vi "write relay.vi"(8 "error in (no error)":errorcluster, 9 "value":bool, 10 "index":i32, 11 "USB DAQ in":refnum<class "USB DAQ.lvclass">) -> (0 "error out":errorcluster, 3 "USB DAQ out":refnum<class "USB DAQ.lvclass">)   [LabVIEW 2025, in "USB DAQ.lvclass"]
uses:
  USB DAQ.lvclass
  USB DAQ.lvclass/USB DAQ.ctl
  <vilib>/DAQmx/write.llb/DAQmx Write (Digital 1D Bool NChan 1Samp 1Line).vi
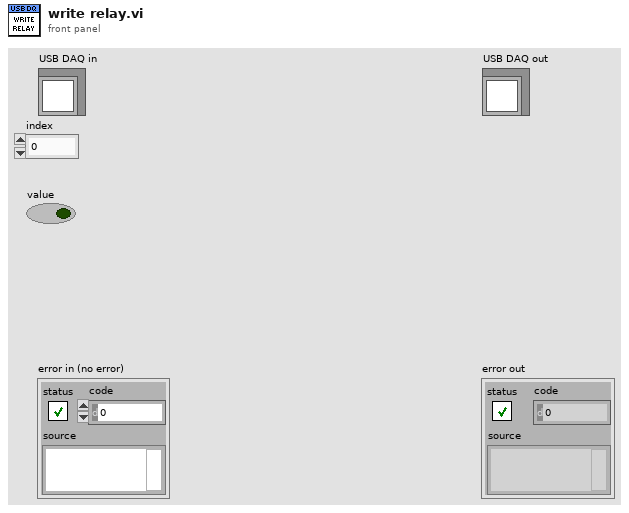
[diagram p1: front panel]
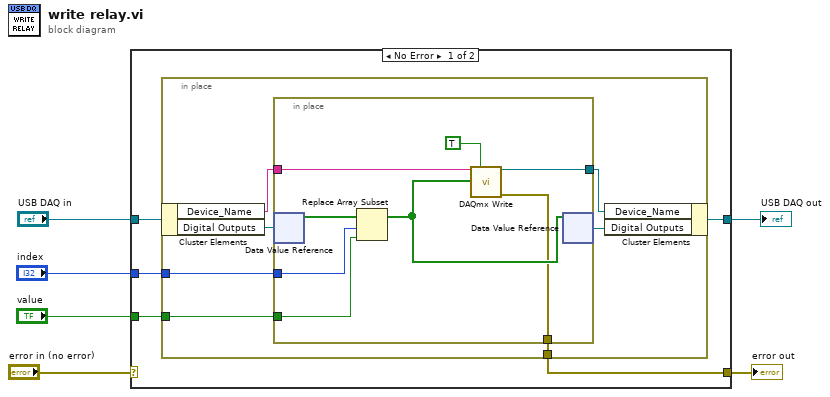
[diagram p0: block diagram]
diagram:
  n1 = case shown="No Error" "error in (no error)" {
    selector: "error in (no error)" -> [_ w28]
    tunnel: [w7 w28] -> w5
    tunnel: [w11 w27] -> w3
    tunnel: "USB DAQ in" -> [w8 w27]
    tunnel: "index" -> [w10 _]
    tunnel: "value" -> [w9 _]
    frame No Error {
      n2 = in-place {
        in-place-border: w10 -> [w16]
        in-place-border: w9 -> [w15]
        in-place-border: [w13] -> w7
        n3 = in-place-cluster #1(w8) -> ("Device_Name"=w14:string, "Digital Outputs"=w18:refnum<data-value>)
        n4 = in-place {
          in-place-border: w16 -> [w25]
          in-place-border: w15 -> [w24]
          in-place-border: w14 -> [w23]
          in-place-border: [w20] -> w13
          in-place-border: [w19] -> w12
          n5 = in-place-dvr #2(w18) -> (w26:bool[])  [unwired: 1 out]
          n6 = Replace Array Subset(array=w26, new element=w24, index=w25) -> (w21:bool[])
          n7 = call-poly <vilib>:"DAQmx Write.vi"("task/channels in"=w23, "auto start"=TRUE, "data"=w21) -> ("task out"=w19:refnum<k21>, "error out"=w20:errorcluster)  [unwired: 10 in, 1 out]
          n8 = in-place-dvr #2(w21) -> (w17:refnum<data-value>)  [unwired: 1 out]
        }
        n9 = in-place-cluster #1("Device_Name"=w12, "Digital Outputs"=w17) -> (w11:refnum<class "USB DAQ.lvclass">)
      }
    }
    frame Error {
    }
  }
  "error out" <- w5
  "USB DAQ out" <- w3
